vi "Demo2 (FPGA).vi"   [LabVIEW 2011]
uses:
  Instance           1 20Saved   Demo2 (FPGA) .vi
  <vilib>/rvi/eio/common/nirviEmuTemplateMethod_errors.vi
  <vilib>/rvi/interface/RandomDataEmulation/nirviRandomDataFPGAFIFO.vi
  <vilib>/rvi/interface/RandomDataEmulation/niFpgaRandomDataHandleErrors.vi
  <vilib>/eio/EIONode/EIONode.xnode
  <vilib>/rvi/DataTransferAndStorage/Container/XNode/niFpgaContainer.xnode
  <vilib>/rvi/interface/RandomDataEmulation/nirviRandomDataFpgaReadWriteTemplate.vi
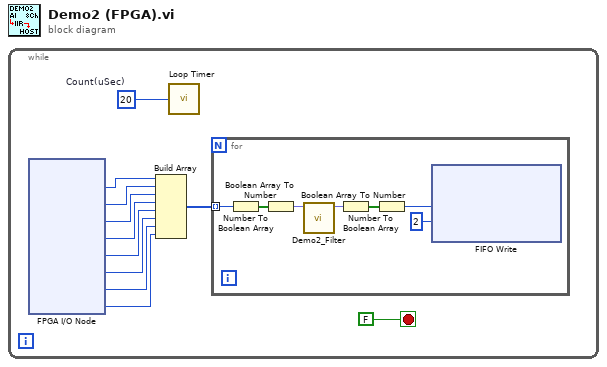
[diagram p0: block diagram]
diagram:
  n1 = while {
    stop <- FALSE stop-if-true
    w1 = u16 20  # Count(uSec)
    n2 = xnode "FPGA I/O Node"() -> ("AI0"=w10:i16, "AI1"=w9:i16, "AI2"=w8:i16, "AI3"=w7:i16, "AI4"=w6:i16, "AI5"=w5:i16, "AI6"=w4:i16, "AI7"=w3:i16)  [unwired: 8 in, 8 out]
    n3 = Build Array(w10, w9, w8, w7, w6, w5, w4, w3) -> (w2:i16[])
    n4 = call "Loop Timer"("Count(uSec)"=w1) -> ()  [unwired: 1 out]
    n5 = for {
      tunnel: w2 -> [w16] mode=indexing
      n6 = Number To Boolean Array(number=w16) -> (Boolean array=w15:bool[])
      n7 = Boolean Array To Number(Boolean array=w15) -> (number=w14:fxp<+/-,16,1>)
      n8 = call "Demo2_Filter.vi"("input data"=w14) -> ("output data"=w18:fxp<+/-,16,5>)  [unwired: 1 in, 9 out]
      n9 = Number To Boolean Array(number=w18) -> (Boolean array=w13:bool[])
      n10 = Boolean Array To Number(Boolean array=w13) -> (number=w12:i16)
      n11 = xnode ("FIFO Write")("Element"=w12, "Timeout"=2) -> ()  [unwired: 1 in, 2 out]
    }
  }
